vi "Finalize.vi"(8 "error in":errorcluster, 11 "shared resources":refnum<class "Shared Resources.lvclass">) -> (0 "error out":errorcluster, 3 "shared resources out":refnum<class "Shared Resources.lvclass">)   [LabVIEW 2020, in "AIM MIL-STD-1553 Engine.lvlib" / "Implementation.lvlib" / "Shared Resources.lvclass"]
uses:
  Shared Resources.lvclass
  Logging/Word Logging/Log Producer/Log Producer.lvclass
  Logging/Word Logging/Word Logging.lvlib
  Hardware API/Module Reference.ctl
  Hardware API/AIM MIL-STD-1553 Hardware API.lvlib
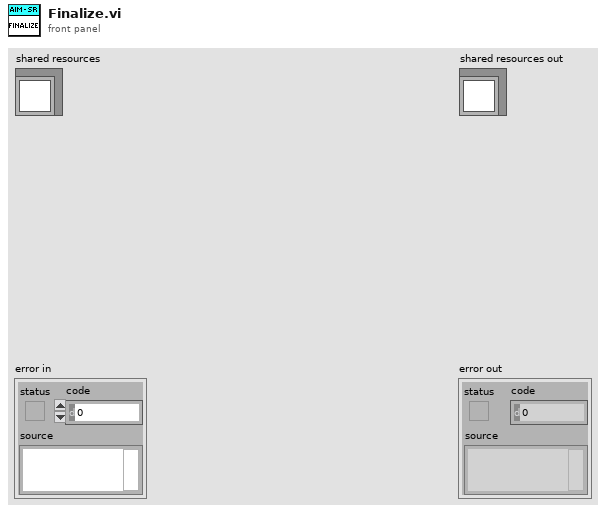
[diagram p1: front panel]
types:
  T1 = typedef "AIM MIL-STD-1553 Hardware API.lvlib/Module Reference.ctl" = u32
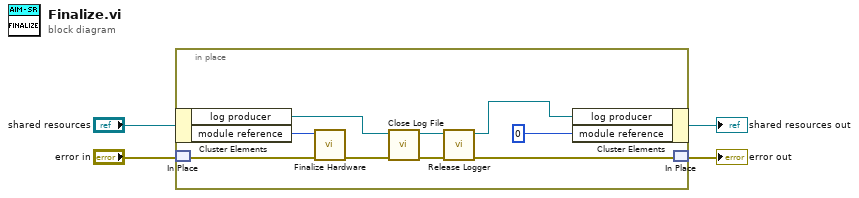
[diagram p0: block diagram]
diagram:
  n1 = in-place {
    n2 = in-place-cluster #1("shared resources") -> ("log producer"=w8:refnum<class "Log Producer.lvclass">, "module reference"=w12:T1)
    n3 = in-place-match #2("error in") -> (w13:errorcluster)
    n4 = call "Finalize Hardware.vi"("error in"=w13, "module reference"=w12) -> ("error out"=w10:errorcluster)  [unwired: 9 in]
    n5 = call "Close Log File.vi"("error in (no error)"=w10, "Log Producer in"=w8) -> ("error out"=w11:errorcluster, "Log Producer out"=w7:refnum<class "Log Producer.lvclass">)  [unwired: 8 in]
    n6 = call "Release Logger.vi"("error in (no error)"=w11, "Producer"=w7) -> ("error out"=w9:errorcluster, "Default Producer"=w6:refnum<class "Log Producer.lvclass">)  [unwired: 8 in]
    n7 = in-place-cluster #1("log producer"=w6, "module reference"=T1 0) -> (→"shared resources out":refnum<class "Shared Resources.lvclass">)
    n8 = in-place-match #2(w9) -> (→"error out":errorcluster)
  }
